vi "Install Octave Package golpi GUI.vi"(8 "error in (no error)":errorcluster, 10 "Verbose? (True)":bool=TRUE, 11 "feature":T1) -> (0 "error out":errorcluster, 3 "Path":path)   [LabVIEW 2020, in "GOLPI library.lvlib"]
uses:
  GOLPI library.lvlib
  Type Definitions/GOLPI package Feature.ctl
  GUI Panel Control Action.ctl
  <vilib>/regexp/Match Regular Expression.xnode
panel:
  out "Instructions:":string
  in  "btn install":bool
  in  "btn cancel":bool
  in  "btn find man":bool
  in  "builds":i32[](listbox) caption="Found GOLPI packages:"
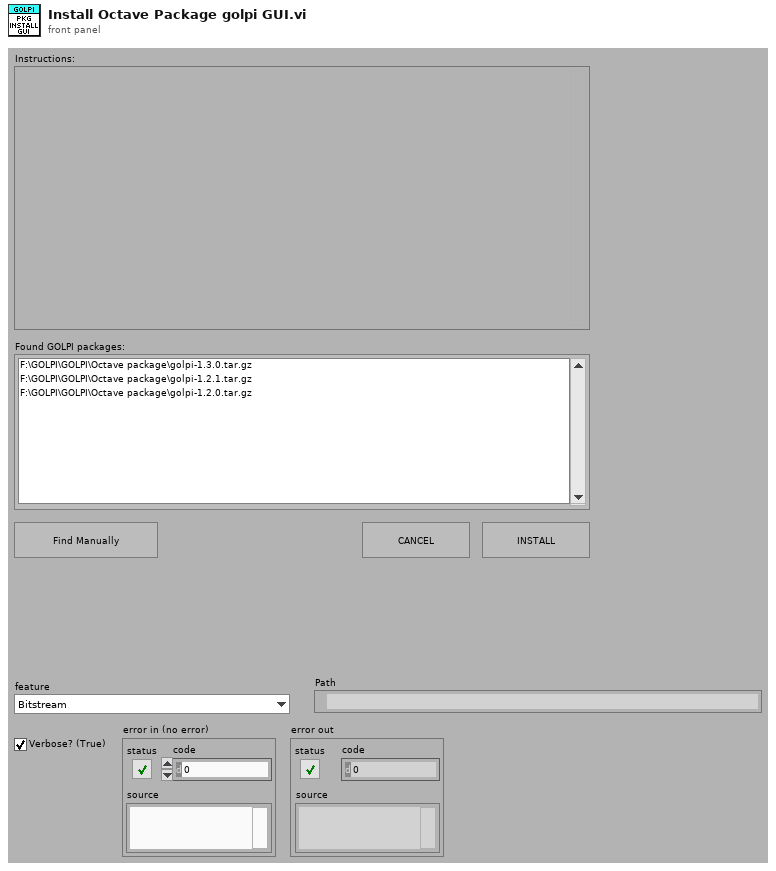
[diagram p1: front panel]
types:
  T1 = typedef "GOLPI package Feature.ctl" = enum16{"Bitstream", "Struct", "Pipes"}
  T2 = typedef "GOLPI library.lvlib/GUI Panel Control Action.ctl" = enum16{"Open hidden", "Open panel", "Close panel", "Bring To Front"}
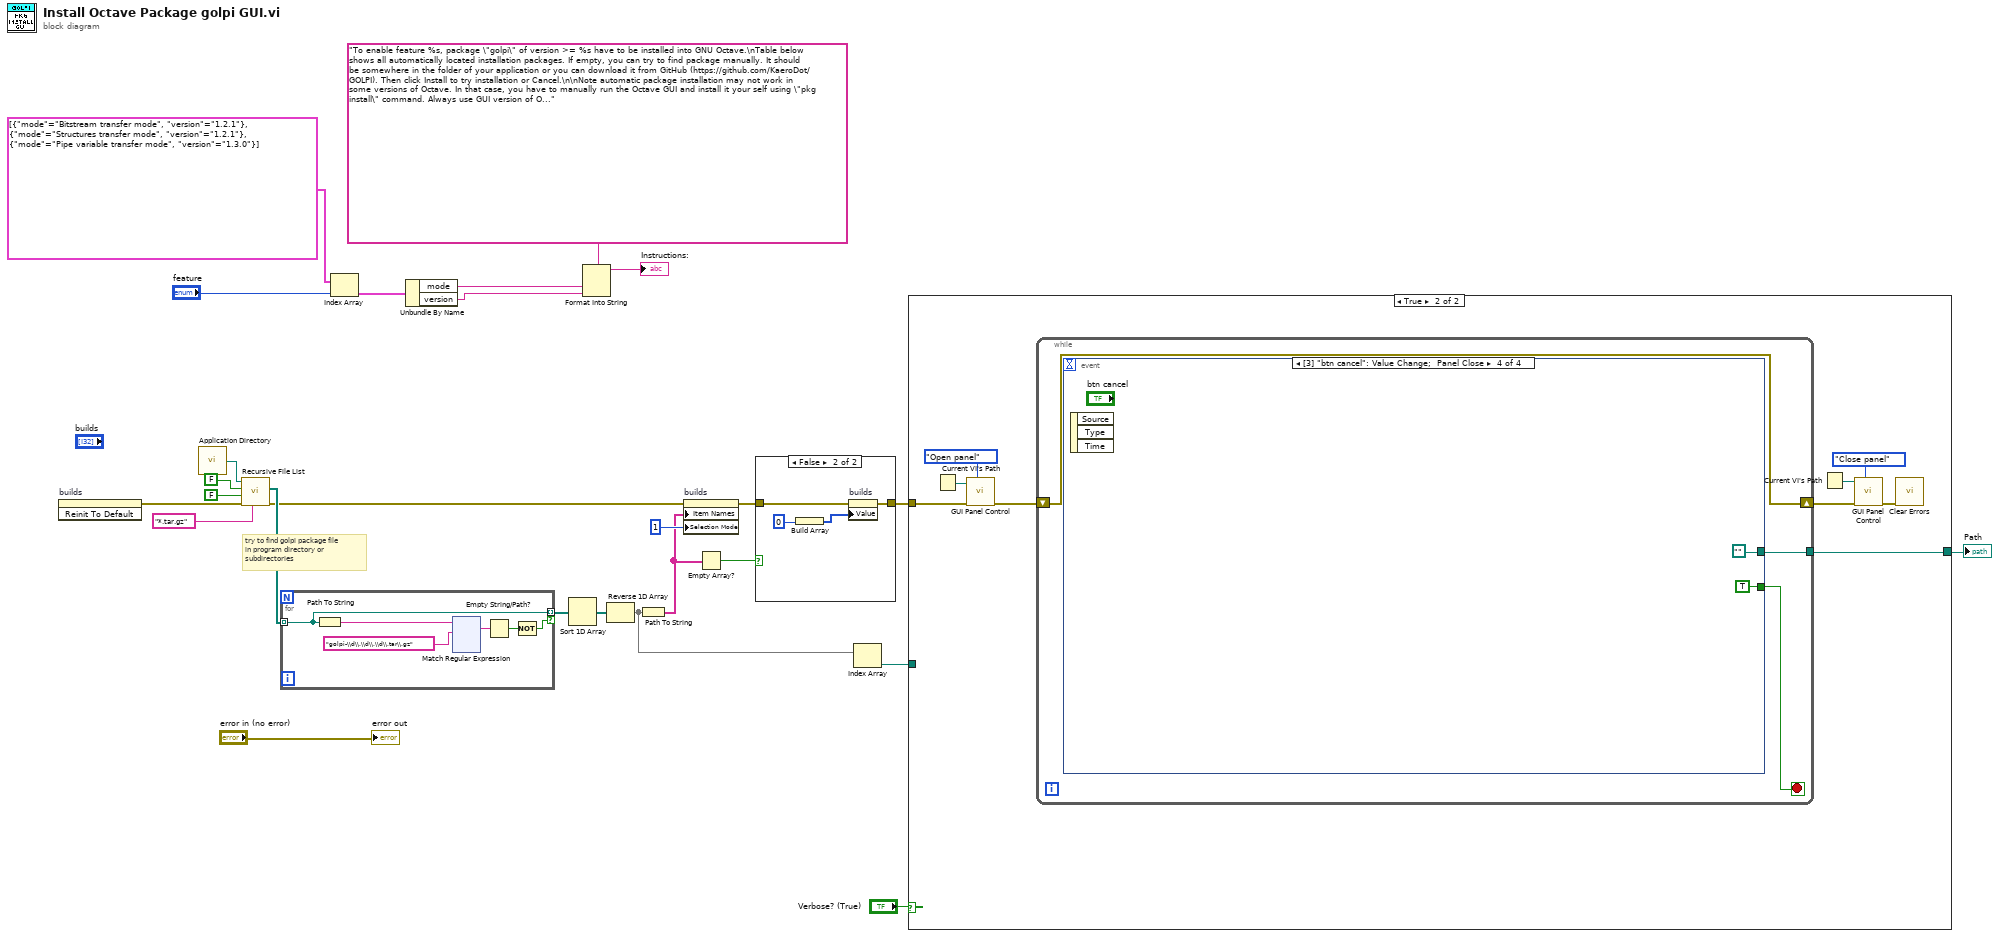
[diagram p0: block diagram]
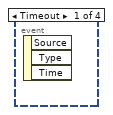
[diagram p3: hidden frame]
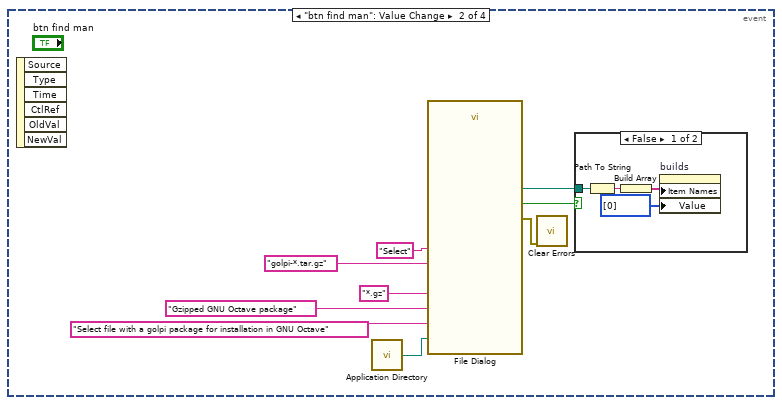
[diagram p4: hidden frame]
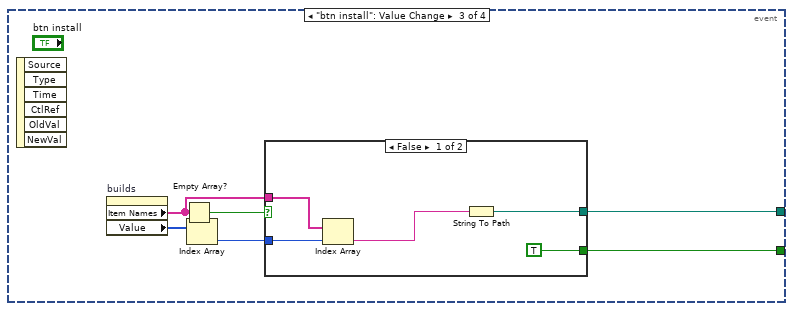
[diagram p6: hidden frame]
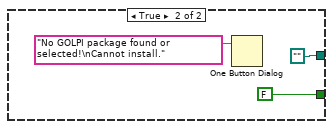
[diagram p7: hidden frame]
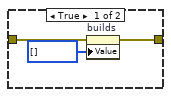
[diagram p8: hidden frame]
diagram:
  # "try to find golpi package file\nin program directory or\nsubdirectories"
  n1 = invoke on="builds" class="LstBox (strict)" method="Reinit To Default"() -> (error out=w19:errorcluster)  [unwired: 3 in, 2 out]
  n2 = call <vilib>:"Application Directory.vi"() -> ("Application Directory"=w26:path)
  n3 = call <vilib>:"Recursive File List.vi"("pattern"="*.tar.gz", "error in (no error)"=w19, "Continue Recursing on Error? (F)"=FALSE, "Treat LLBs as Folders?"=FALSE, "Folder Path"=w26) -> ("error out"=w18:errorcluster, "All Files in Dir"=w25:path[])  [unwired: 2 in, 3 out]
  n4 = for {
    tunnel: w25 -> [w29] mode=indexing
    tunnel: [w29] -> w24 mode=indexing if=w28
    n5 = Path To String(path=w29) -> (string=w27:string)
    n6 = xnode "Match Regular Expression"("input string"=w27, "regular expression"="golpi-\\d\\.\\d\\.\\d\\.tar\\.gz") -> ("whole match"=w31:string)  [unwired: 4 in, 4 out]
    n7 = Empty String/Path?(string/path=w31) -> (empty?=w30:bool)
    n8 = Not(x=w30) -> (.not. x?=w28:bool)
  }
  n9 = Index Array(array=cluster{"mode":string, "version":string}[] [{"mode"="Bitstream transfer mode", "version"="1.2.1"}, {"mode"="Structures transfer mode", "version"="1.2.1"}, {"mode"="Pipe variable transfer mode", "version"="1.3.0"}], index="feature") -> (element=w9:cluster{"mode":string, "version":string})
  n10 = Unbundle By Name(w9) -> ("mode"=w8:string, "version"=w7:string)
  n11 = Sort 1D Array(array=w24) -> (sorted array=w23:path[])
  n12 = Format Into String(format string="To enable feature %s, package \"golpi\" of version >= %s have to be installed into GNU Octave.\nTable below shows all automatically located installation packages. If empty, you can try to find package manually. It should be somewhere in the folder of your application or you can download it from GitHub (https://github.com/KaeroDot/GOLPI). Then click Install to try installation or Cancel.\n\nNote automatic package installation may not work in some versions of Octave. In that case, you have to manually run the Octave GUI and install it your self using \"pkg install\" command. Always use GUI version of Octave, not console one as it is a bit buggy. You can start Octave GUI from Windows Start menu. Also make sure you select the same version of Octave as you have selected in LabVIEW as you may have several versions installed and packages are installed individually for each version! \n\nIf, for some reason, Octave fails to compile *.oct files (error message will be something like \"failed .CONFIGURE script\"), you may install older GOLPI package version 1.2.1 (also included). In this case, you won't be able to use pipe variable transfer mode, but bitstream and structures transfer modes will work." ("message"), w8, w7) -> (resulting string=→"Instructions:":string)  [unwired: 2 in, 1 out]
  n13 = Reverse 1D Array(array=w23) -> (reversed array=w5:path[])
  n14 = Path To String(path=w5) -> (string=w16:string[])
  n15 = property on="builds" class="LstBox (strict)"(error in=w18, "Item Names"=w16, "Selection Mode"=1) -> (error out=w14:errorcluster)  [unwired: 1 in, 1 out]
  n16 = Empty Array?(array=w16) -> (empty?=w15:bool)
  n17 = case shown="False" w15 {
    tunnel: w14 -> [w149 w153]
    tunnel: [w147 w152] -> w13
    frame True {
      n18 = property on="builds" class="LstBox (strict)"(error in=w149, "Value"=i32[] [] ("builds")) -> (error out=w147:errorcluster)  [unwired: 1 in, 1 out]
    }
    frame False {
      n19 = Build Array(0) -> (w150:i32[])
      n20 = property on="builds" class="LstBox (strict)"(error in=w153, "Value"=w150) -> (error out=w152:errorcluster)  [unwired: 1 in, 1 out]
    }
  }
  n21 = Index Array(array=w5) -> (element=w1:path)  [unwired: 1 in]
  n22 = case shown="True" "Verbose? (True)" {
    tunnel: w13 -> [_ w161]
    tunnel: [w154 w163] -> w2
    tunnel: w1 -> [w154 _]
    frame False {
    }
    frame True {
      n23 = Current VI's Path() -> (path=w158:path)
      n24 = call "GUI Panel Control.vi"("action (open panel)"=GUI_Panel_Control_Action."Open panel", "error in (no error)"=w161, "vi path"=w158) -> ("error out"=w160:errorcluster)  [unwired: 8 in]
      n25 = while {
        tunnel: [w165] -> w163
        shift-right: [w164] -> w159
        shift-left: w160 -> [w164]
        stop <- w166 stop-if-true
        n26 = event shown="[3] \"btn cancel\": Value Change;  Panel Close" {
          selector: _ -> [_ _ _ _]
          dyn-events: _ -> [_ _ _ _]
          timeout: _ -> [_ _ _ _]
          tunnel: [_ _ w183 TRUE] -> w166
          tunnel: [_ _ w180 path ""] -> w165
          event Timeout {
            n27 = event-data() -> ()  [unwired: 1 in, 3 out]
          }
          event "btn find man": Value Change {
            n28 = event-data() -> ()  [unwired: 1 in, 6 out]
            n29 = call <vilib>:"Application Directory.vi"() -> ("Application Directory"=w170:path)
            n30 = call "File Dialog"("start path"=w170, "prompt"="Select file with a golpi package for installation in GNU Octave", "button label"="Select", "default name"="golpi-*.tar.gz", "pattern (all files)"="*.gz", "pattern label"="Gzipped GNU Octave package") -> ("selected path"=w167:path, "cancelled"=w168:bool, "error out"=w169:errorcluster)  [unwired: 6 in, 1 out]
            n31 = call <vilib>:"Clear Errors.vi"("error in (no error)"=w169) -> ()  [unwired: 5 in, 2 out]
            n32 = case shown="False" w168 {
              tunnel: w167 -> [w179 _]
              frame False {
                n33 = Path To String(path=w179) -> (string=w178:string)
                n34 = Build Array(w178) -> (w177:string[])
                n35 = property on="builds" class="LstBox (strict)"("Item Names"=w177, "Value"=i32[] [0] ("builds")) -> ()  [unwired: 2 in, 2 out]
              }
              frame True {
              }
            }
          }
          event "btn install": Value Change {
            n36 = event-data() -> ()  [unwired: 1 in, 6 out]
            n37 = property on="builds" class="LstBox (strict)"() -> ("Item Names"=w181:string[], "Value"=w185:i32[])  [unwired: 2 in, 2 out]
            n38 = Empty Array?(array=w181) -> (empty?=w184:bool)
            n39 = Index Array(array=w185) -> (element=w182:i32)  [unwired: 1 in]
            n40 = case shown="False" w184 {
              tunnel: [TRUE FALSE] -> w183
              tunnel: w182 -> [w189 _]
              tunnel: w181 -> [w188 _]
              tunnel: [w186 path ""] -> w180
              frame False {
                n41 = Index Array(array=w188, index=w189) -> (element=w187:string)
                n42 = String To Path(string=w187) -> (path=w186:path)
              }
              frame True {
                n43 = One Button Dialog(message="No GOLPI package found or selected!\nCannot install.") -> ()  [unwired: 1 in, 1 out]
              }
            }
          }
          event "btn cancel": Value Change; Panel Close {
            n44 = event-data() -> ()  [unwired: 1 in, 3 out]
          }
        }
      }
      n45 = Current VI's Path() -> (path=w157:path)
      n46 = call "GUI Panel Control.vi"("action (open panel)"=GUI_Panel_Control_Action."Close panel", "error in (no error)"=w159, "vi path"=w157) -> ("error out"=w156:errorcluster)  [unwired: 8 in]
      n47 = call <vilib>:"Clear Errors.vi"("error in (no error)"=w156) -> ()  [unwired: 5 in, 2 out]
    }
  }
  "Path" <- w2
  "error out" <- "error in (no error)"
